vi "AxisRanges.vi"(0 "x":dbl[][](array[numeric]) format="%.2f", 5 "y":dbl[][](array[numeric]) format="%.4f", 9 "# rf points per line":u16, 11 "# lines per scan":u16) -> (3 "X right":dbl format="%.2f", 4 "X left":dbl format="%.2e", 6 "X step":dbl format="%.2e", 10 "Y low":dbl format="%.4e", 14 "Y high":dbl format="%.2f", 15 "Y step":dbl format="%.2e")   [LabVIEW 2022 SP3]
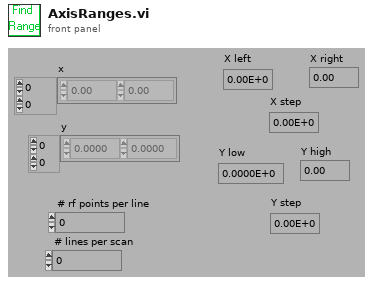
[diagram p1: front panel]
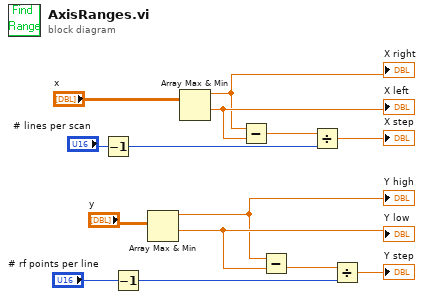
[diagram p0: block diagram]
diagram:
  n1 = Decrement(x="# lines per scan") -> (x-1=w1:u16)
  n2 = Decrement(x="# rf points per line") -> (x-1=w2:u16)
  n3 = Array Max & Min(array="y") -> (max value=w10:dbl, min value=w11:dbl)  [unwired: 2 out]
  "Y low" <- w11
  "Y high" <- w10
  n4 = Array Max & Min(array="x") -> (max value=w12:dbl, min value=w13:dbl)  [unwired: 2 out]
  "X left" <- w13
  "X right" <- w12
  n5 = Subtract(x=w12, y=w13) -> (x-y=w3:dbl)
  n6 = Subtract(x=w10, y=w11) -> (x-y=w4:dbl)
  n7 = Divide(x=w3, y=w1) -> (x/y=→"X step":dbl)
  n8 = Divide(x=w4, y=w2) -> (x/y=→"Y step":dbl)
